vi "GEOM_GetValueFromInfo.vi"(9 "Key":string, 10 "Info":string[][](table)) -> (1 "found?":bool, 2 "Value":string)   [LabVIEW 2016]
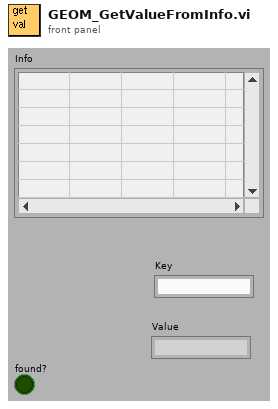
[diagram p1: front panel]
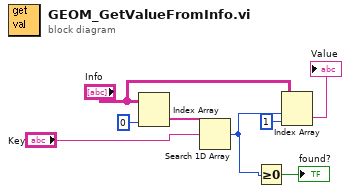
[diagram p0: block diagram]
diagram:
  n1 = Index Array(array="Info", index (col)=0 ("disabled index (col)")) -> (element=w7:string[])  [unwired: 1 in]
  n2 = Search 1D Array(1D array=w7, element="Key") -> (index of element=w4:i32)  [unwired: 1 out]
  n3 = Greater Or Equal To 0?(x=w4) -> (x >= 0?=→"found?":bool)
  n4 = Index Array(array="Info", index (row)=w4, index (col)=1 ("disabled index (col)")) -> (element=→"Value":string)
